vi "Read Clock Discipline.vi"(8 "error in (no error)":errorcluster, 11 "RT Data Cluster in":T1={"Timekeeper hdl"="", "clkDisc session"=variant, "Compiled Data"={"SyncMod?"=FALSE, "SyncMod"="", "ConnectionSettings"={"Mode"=enum."Generate sample clock", "pxitrig"=FALSE, "pfi0"=FALSE, "pfi1"=FALSE, "pfi2"=FALSE, "External Pin"=enum."PFI0", "Routes"=[]}, "TimeKeeper"="", "ScanOffset(%)"=0.0, "StartDelay(s)"=0, "Time Ref Settings"={"Time Reference"=enum."GPS", "Priority 1"=0, "Priority 2"=0, "IRIG type"=enum."IRIGB AM", "Terminal"="", "PPSSetTime"=FALSE, "Start Time"=timestamp(0 s since 1904-01-01)}, "FIFO Locations"={"SysTime"=[], "TimeRef"=[], "Status"=[]}}, "OutputsData"=[], "OutputsFIFO"=refnum, "Scan Period"=0, "Timekeeper type"=enum."6683", "SyncMod type"=enum."6683", "SyncMod hdl"=""} {"Compiled Data"."Time Ref Settings"."Priority 2" min=0 max=255; "Compiled Data"."Time Ref Settings"."Priority 1" min=0 max=255}) -> (0 "error out":errorcluster, 3 "RT Data Cluster out":T1={"Timekeeper hdl"="", "clkDisc session"=variant, "Compiled Data"={"SyncMod?"=FALSE, "SyncMod"="", "ConnectionSettings"={"Mode"=enum."Generate sample clock", "pxitrig"=FALSE, "pfi0"=FALSE, "pfi1"=FALSE, "pfi2"=FALSE, "External Pin"=enum."PFI0", "Routes"=[]}, "TimeKeeper"="", "ScanOffset(%)"=0.0, "StartDelay(s)"=0, "Time Ref Settings"={"Time Reference"=enum."GPS", "Priority 1"=0, "Priority 2"=0, "IRIG type"=enum."IRIGB AM", "Terminal"="", "PPSSetTime"=FALSE, "Start Time"=timestamp(0 s since 1904-01-01)}, "FIFO Locations"={"SysTime"=[], "TimeRef"=[], "Status"=[]}}, "OutputsData"=[], "OutputsFIFO"=refnum, "Scan Period"=0, "Timekeeper type"=enum."6683", "SyncMod type"=enum."6683", "SyncMod hdl"=""} {"Compiled Data"."Time Ref Settings"."Priority 2" min=0 max=255; "Compiled Data"."Time Ref Settings"."Priority 1" min=0 max=255}, 5 "Sync":bool)   [LabVIEW 2015, in "Chassis TimeSync Engine.lvlib"]
uses:
  Chassis TimeSync Engine.lvlib
  RT Data Cluster.ctl
  mdevClkDisc.llb/_clkDisc_session.ctl
  Shared/Compiled Data.ctl
  Shared/Connection Settings.ctl
  Shared/Mode.ctl
  Shared/External Pin.ctl
  Shared/Routes.ctl
  Shared/Route.ctl
  Shared/Time Ref Settings.ctl
  Shared/Time Reference.ctl
  Shared/IRIG Type.ctl
  timekeeper type.ctl
  Shared/Chassis TimeSync Shared.lvlib
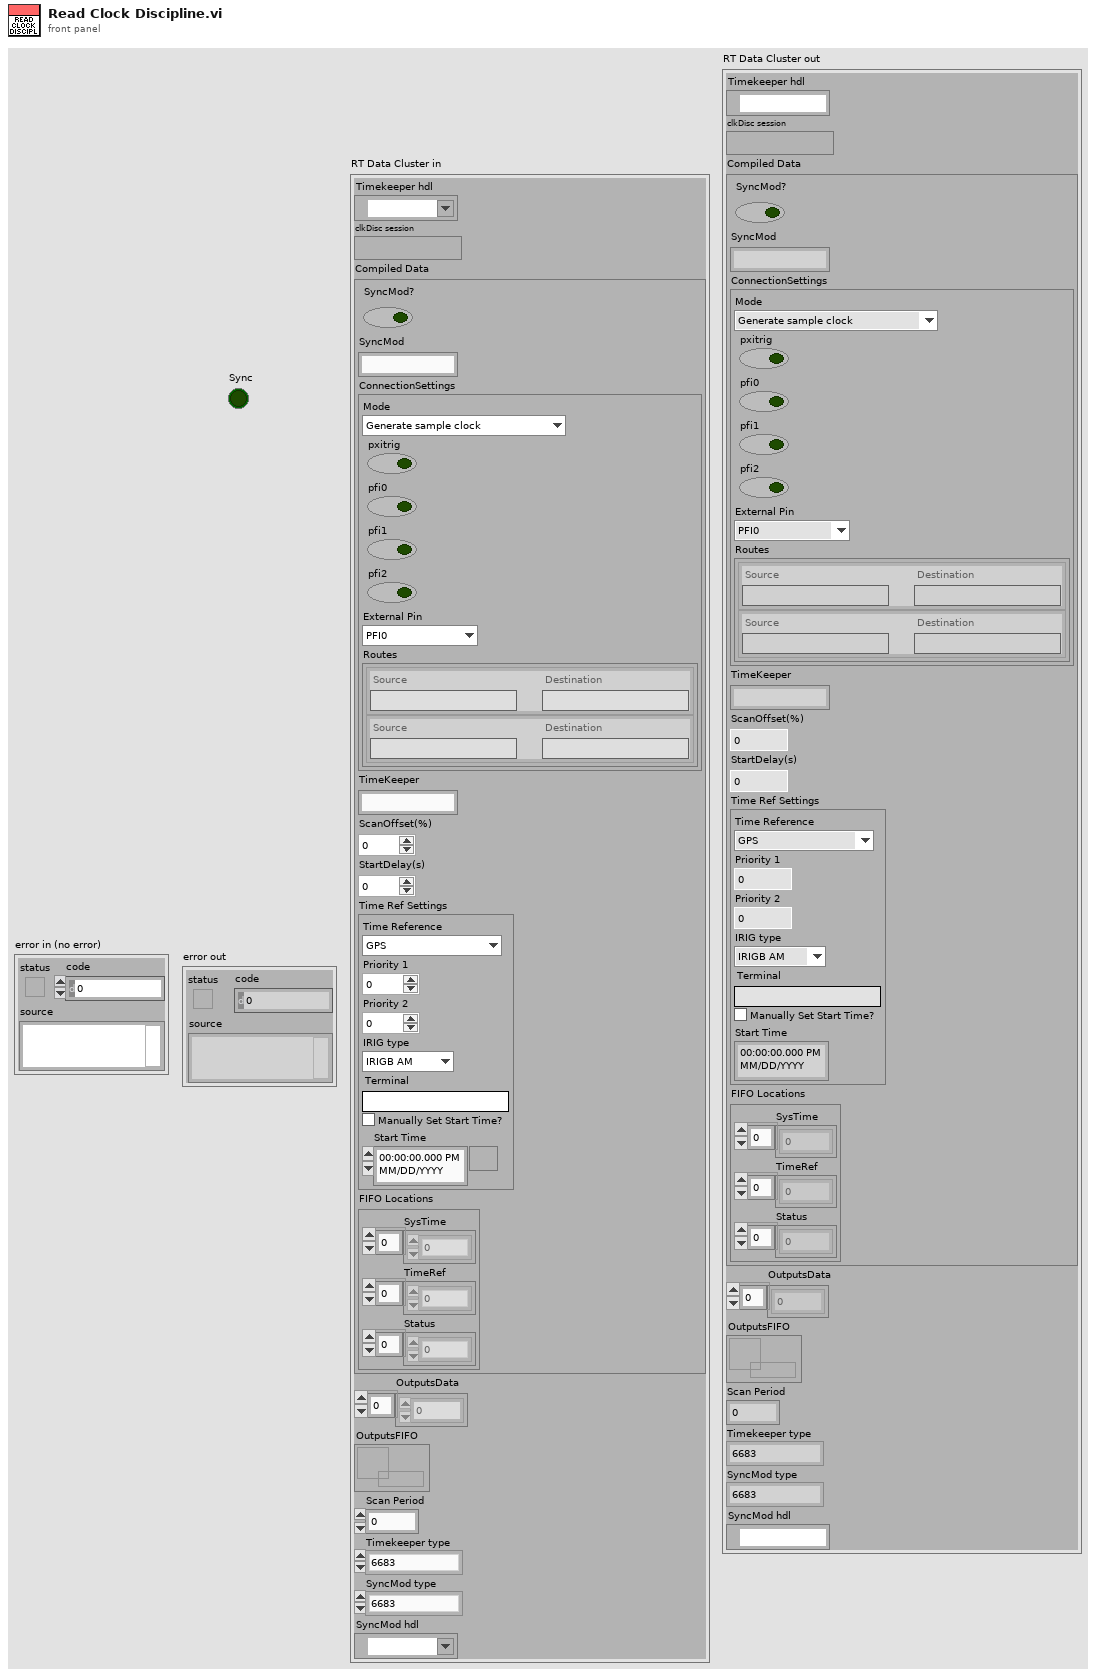
[diagram p1: front panel]
types:
  T1 = typedef "Chassis TimeSync Engine.lvlib/RT Data Cluster.ctl" = cluster{"Timekeeper hdl":refnum<k15>, "clkDisc session":T2, "Compiled Data":T3, "OutputsData":dbl[], "OutputsFIFO":refnum<k33>, "Scan Period":u32, "Timekeeper type":T12, "SyncMod type":T12, "SyncMod hdl":refnum<k15>}
  T2 = typedef "_clkDisc_session.ctl" = variant
  T3 = typedef "Chassis TimeSync Shared.lvlib/Compiled Data.ctl" = cluster{"SyncMod?":bool, "SyncMod":string, "ConnectionSettings":T4, "TimeKeeper":string, "ScanOffset(%)":dbl, "StartDelay(s)":u16, "Time Ref Settings":T9, "FIFO Locations":cluster{"SysTime":i32[], "TimeRef":i32[], "Status":i32[]}}
  T4 = typedef "Chassis TimeSync Shared.lvlib/Connection Settings.ctl" = cluster{"Mode":T5, "pxitrig":bool, "pfi0":bool, "pfi1":bool, "pfi2":bool, "External Pin":T6, "Routes":T7}
  T5 = typedef "Chassis TimeSync Shared.lvlib/Mode.ctl" = enum16{"Generate sample clock", "Route sample clock out of chassis", "Route sample clock into chassis", "Custom routes"}
  T6 = typedef "Chassis TimeSync Shared.lvlib/External Pin.ctl" = enum16{"PFI0", "PFI1", "PFI2"}
  T7 = typedef "Chassis TimeSync Shared.lvlib/Routes.ctl" = T8[]
  T8 = typedef "Chassis TimeSync Shared.lvlib/Route.ctl" = cluster{"Source":string, "Destination":string}
  T9 = typedef "Chassis TimeSync Shared.lvlib/Time Ref Settings.ctl" = cluster{"Time Reference":T10, "Priority 1":i32, "Priority 2":i32, "IRIG type":T11, "Terminal":string, "PPSSetTime":bool, "Start Time":timestamp}
  T10 = typedef "Chassis TimeSync Shared.lvlib/Time Reference.ctl" = enum16{"GPS", "IRIG", "PPS", "1588 Ordinary Clock", "PXI Chassis Clock", "Free Running (Internal)"}
  T11 = typedef "Chassis TimeSync Shared.lvlib/IRIG Type.ctl" = enum16{"IRIGB DC", "IRIGB AM"}
  T12 = typedef "Chassis TimeSync Engine.lvlib/timekeeper type.ctl" = enum16{"6683", "6683H", "6682", "6682H", "non-timekeeper", "timekeeper"}
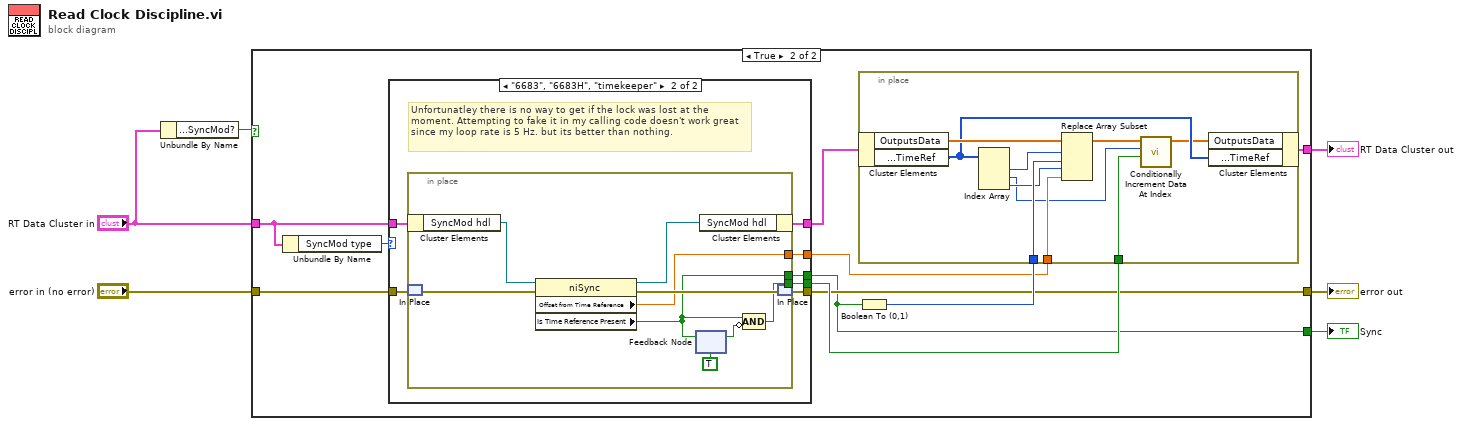
[diagram p0: block diagram]
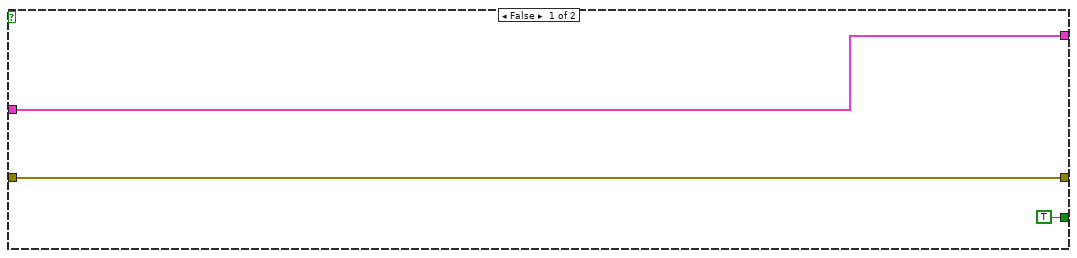
[diagram p2: hidden frame]
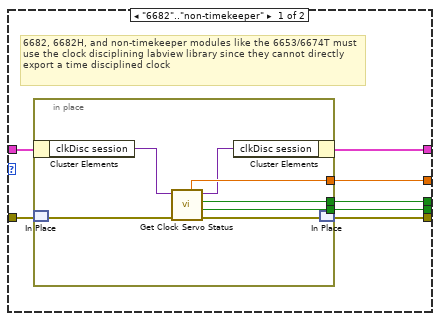
[diagram p3: hidden frame]
diagram:
  n1 = Unbundle By Name("RT Data Cluster in") -> ("Compiled Data.SyncMod?"=w2:bool)
  n2 = case shown="True" w2 {
    tunnel: [w8 w19] -> w6
    tunnel: "error in (no error)" -> [w9 w15]
    tunnel: [w9 w13] -> w4
    tunnel: "RT Data Cluster in" -> [w8 w11]
    tunnel: [TRUE ("Servo Locked") w12] -> w1
    frame False {
    }
    frame True {
      n3 = Unbundle By Name(w11) -> ("SyncMod type"=w10:T12)
      n4 = case shown="\"6683\", \"6683H\", \"timekeeper\"" w10 {
        tunnel: [w26 w40] -> w17
        tunnel: [w25 w39] -> w16
        tunnel: w15 -> [w24 w38]
        tunnel: [w23 w37] -> w14
        tunnel: [w22 w36] -> w13
        tunnel: [w21 w35] -> w12
        tunnel: w11 -> [w20 w34]
        frame "6682".."non-timekeeper" {
          # "6682, 6682H, and non-timekeeper modules like the 6653/6674T must use the clock disciplining labview library since they cannot directly export a time disciplined clock"
          n5 = in-place {
            in-place-border: [w33] -> w21
            in-place-border: [w32] -> w26
            in-place-border: [w31] -> w25
            n6 = in-place-cluster #1(w20) -> ("clkDisc session"=w28:T2)
            n7 = in-place-match #2(w24) -> (w30:errorcluster)
            n8 = call "Get Clock Servo Status.vi"("clkDisc session (in)"=w28, "error out"=w30) -> ("Calculated Time Reference Offset"=w31:dbl, "clkDisc session (out)"=w27:T2, "Servo Locked"=w33:bool, "Servo Lock Lost"=w32:bool, "error (out)"=w29:errorcluster)  [unwired: 2 in]
            n9 = in-place-cluster #1("clkDisc session"=w27) -> (w23:T1)
            n10 = in-place-match #2(w29) -> (w22:errorcluster)
          }
        }
        frame "6683", "6683H", "timekeeper" {
          # "Unfortunatley there is no way to get if the lock was lost at the moment. Attempting to fake it in my calling code doesn't work great since my loop rate is 5 Hz. but its better than nothing."
          n11 = in-place {
            in-place-border: [w42] -> w35
            in-place-border: [w41] -> w40
            in-place-border: [w45] -> w39
            n12 = in-place-cluster #3(w34) -> ("SyncMod hdl"=w48:refnum<k15>)
            n13 = in-place-match #4(w38) -> (w49:errorcluster)
            n14 = property class="niSync"(reference=w48, error in=w49) -> (reference out=w47:refnum<k15>, error out=w46:errorcluster, "Offset from Time Reference"=w45:dbl, "Is Time Reference Present"=w42:bool)
            n15 = feedback-in #5(w42) -> ()
            n16 = feedback #5(TRUE) -> (w43:bool)
            n17 = in-place-cluster #3("SyncMod hdl"=w47) -> (w37:T1)
            n18 = Compound Arithmetic op=AND(w42, invert w43) -> (w41:bool)
            n19 = in-place-match #4(w46) -> (w36:errorcluster)
          }
        }
      }
      n20 = Boolean To (0,1)(Boolean=w12) -> (0, 1=w18:i16)
      n21 = in-place {
        in-place-border: w16 -> [w55]
        in-place-border: w18 -> [w56]
        in-place-border: w17 -> [w50]
        n22 = in-place-cluster #6(w14) -> ("OutputsData"=w59:dbl[], "Compiled Data.FIFO Locations.TimeRef"=w57:i32[])
        n23 = Index Array(array=w57) -> (element #1=w58:i32, element #2=w51:i32, element #3=w54:i32)  [unwired: 3 in]
        n24 = Replace Array Subset(array=w59, new element #1=w56, index #1=w58, new element #2=w55, index #2=w54) -> (w53:dbl[])
        n25 = call "Conditionally Increment Data At Index.vi"("Increment"=w50, "Data index"=w51, "Data in"=w53) -> ("Data out"=w52:dbl[])  [unwired: 8 in]
        n26 = in-place-cluster #6("OutputsData"=w52, "Compiled Data.FIFO Locations.TimeRef"=w57) -> (w19:T1)
      }
    }
  }
  "error out" <- w4
  "RT Data Cluster out" <- w6
  "Sync" <- w1
